vi "case test.vi"() -> ()   [LabVIEW 2016]
panel:
  out "subarray 2":dbl[](array[numeric])
  out "subarray":dbl[](array[numeric])
  in  "Array 2":dbl[][](array[numeric])
  in  "milliseconds to wait":u32
  out "element":dbl
  out "appended array":dbl[](array[numeric])
  in  "Array":dbl[](array[numeric])
  in  "Boolean 2":bool
  out "Boolean 5":bool
  out "Boolean 4":bool
  out "Boolean 3":bool
  in  "Boolean":bool
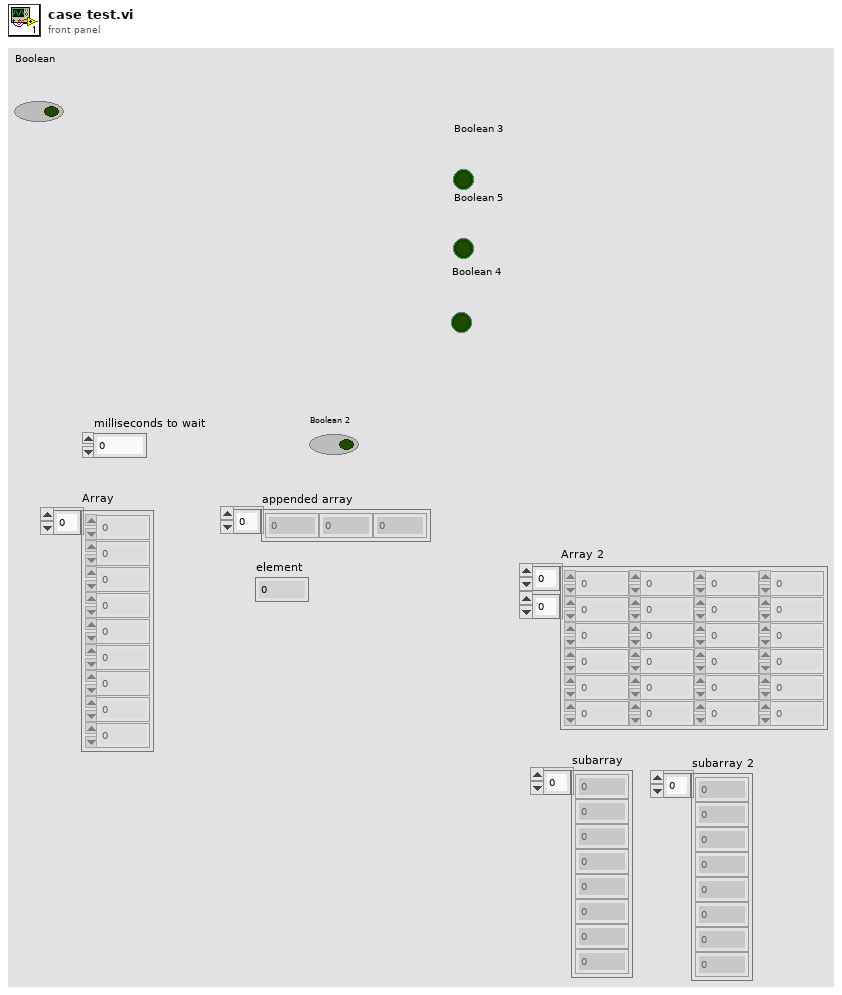
[diagram p1: front panel]
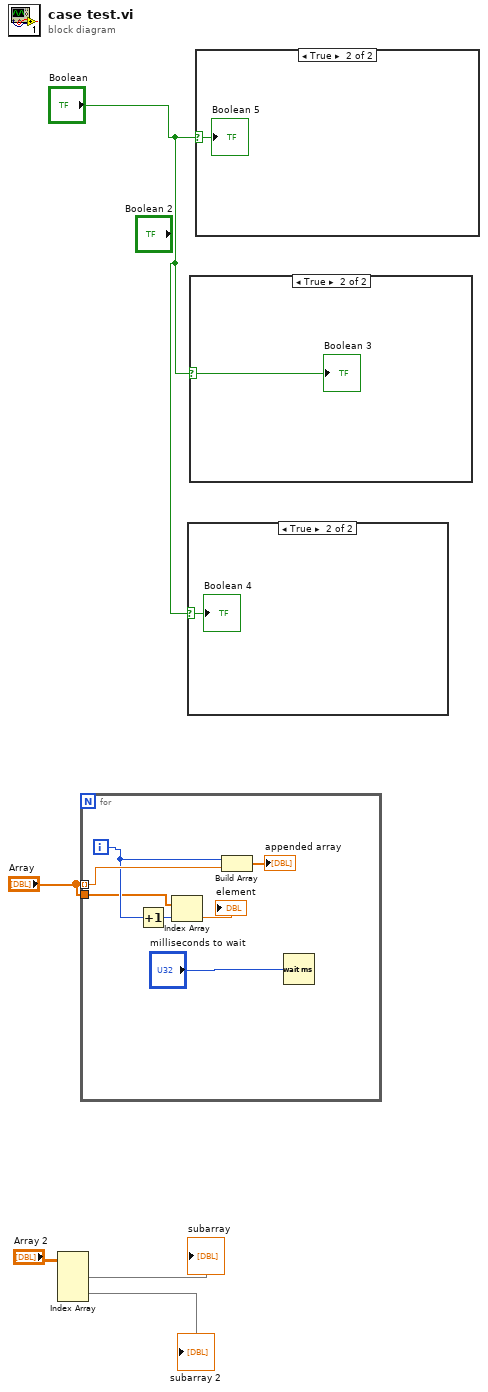
[diagram p0: block diagram]
diagram:
  n1 = Index Array(array="Array 2") -> (element #1=→"subarray":dbl[], element #2=→"subarray 2":dbl[])  [unwired: 4 in]
  n2 = for {
    tunnel: "Array" -> [w12] mode=indexing
    tunnel: "Array" -> [w8]
    i -> [w10]
    n3 = Increment(x=w10) -> (x+1=w9:i32)
    n4 = Index Array(array=w8, index=w9) -> (element=→"element":dbl)
    n5 = Build Array(w10, w12) -> (→"appended array":dbl[])
    n6 = Wait (ms)(milliseconds to wait="milliseconds to wait") -> ()  [unwired: 1 out]
  }
  n7 = case shown="True" "Boolean" {
    selector: "Boolean" -> [_ w13]
    frame False {
    }
    frame True {
      "Boolean 4" <- w13
    }
  }
  n8 = case shown="True" "Boolean" {
    selector: "Boolean" -> [_ w14]
    frame False {
    }
    frame True {
      "Boolean 3" <- w14
    }
  }
  n9 = case shown="True" "Boolean" {
    selector: "Boolean" -> [_ w15]
    frame False {
    }
    frame True {
      "Boolean 5" <- w15
    }
  }
